vi "WFDC Get Current Drift.vi"(0 "Ref Images":T1[](array[typedef]), 2 "Z Calibration (slope, inter)":dbl[](array[numeric]), 5 "Half Shift":i32=7, 7 "Current Image":u16[][](array[numeric]), 11 "Error In":errorcluster, 13 "Track XY Drift?":bool=TRUE) -> (4 "Axis 1 Drift (px)":dbl, 6 "Axis 2 Drift (px)":dbl, 8 "Z Position (µm)":dbl format="%#_10g", 15 "Error Out":errorcluster)   [LabVIEW 2020]
uses:
  <vilib>/vision/Image Controls.llb/IMAQ Image.ctl
  WFDC DLL and Testing/Visual Studio NCC Max Shift DLL/x64/Release/VSmaxShiftNCC.dll
panel:
  out "Fit Middle Corr Image":dbl[][](graph)
  out "Middle Corr Image":dbl[][](graph)
  in  "Ref Image Pixel Size (µm)":dbl
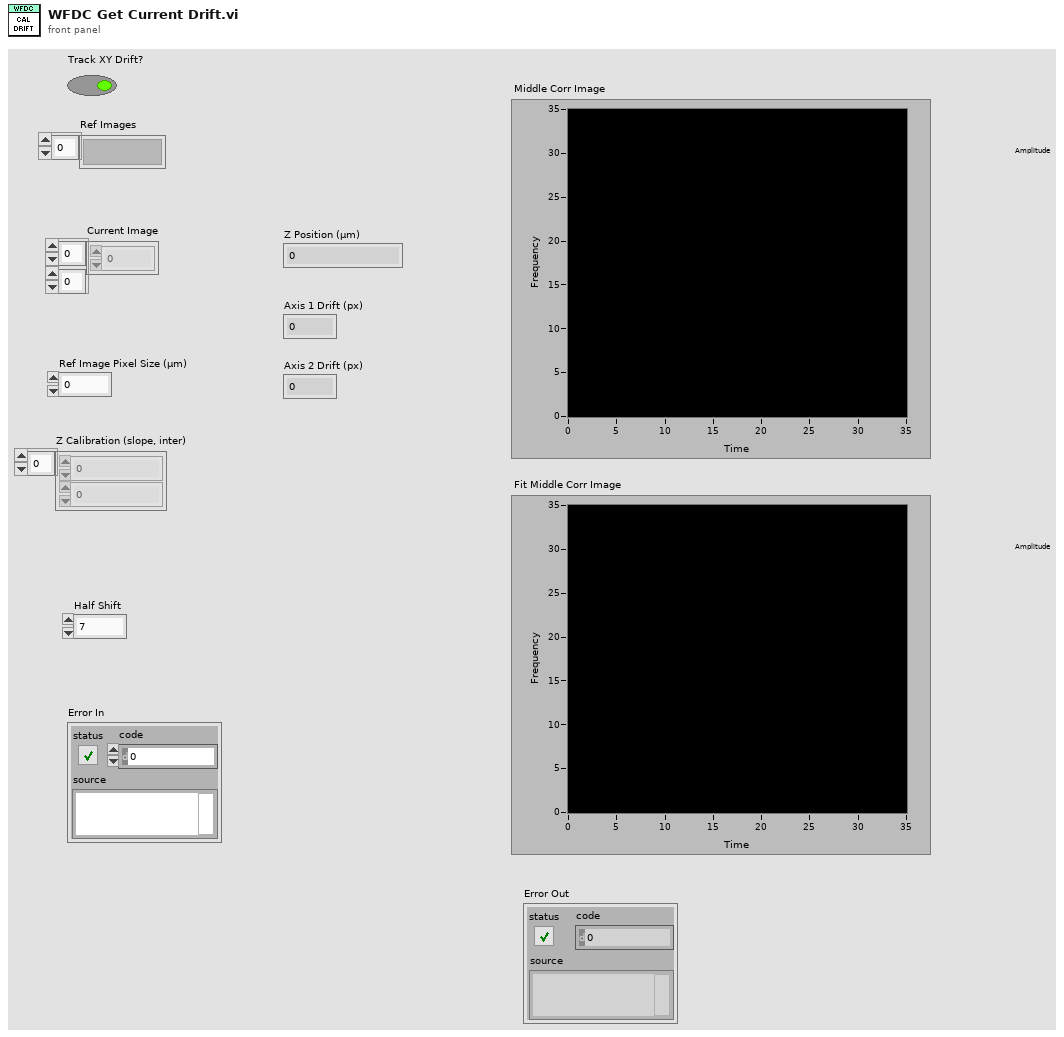
[diagram p1: front panel]
types:
  T1 = typedef "IMAQ Image.ctl" = refnum<image>
  T2 = typedef "2D Gaussian - Best Fit Parameters.ctl" = cluster{"Amplitude":dbl, "X Position":dbl, "Y Position":dbl, "X Width":dbl, "Y Width":dbl, "Offset":dbl}
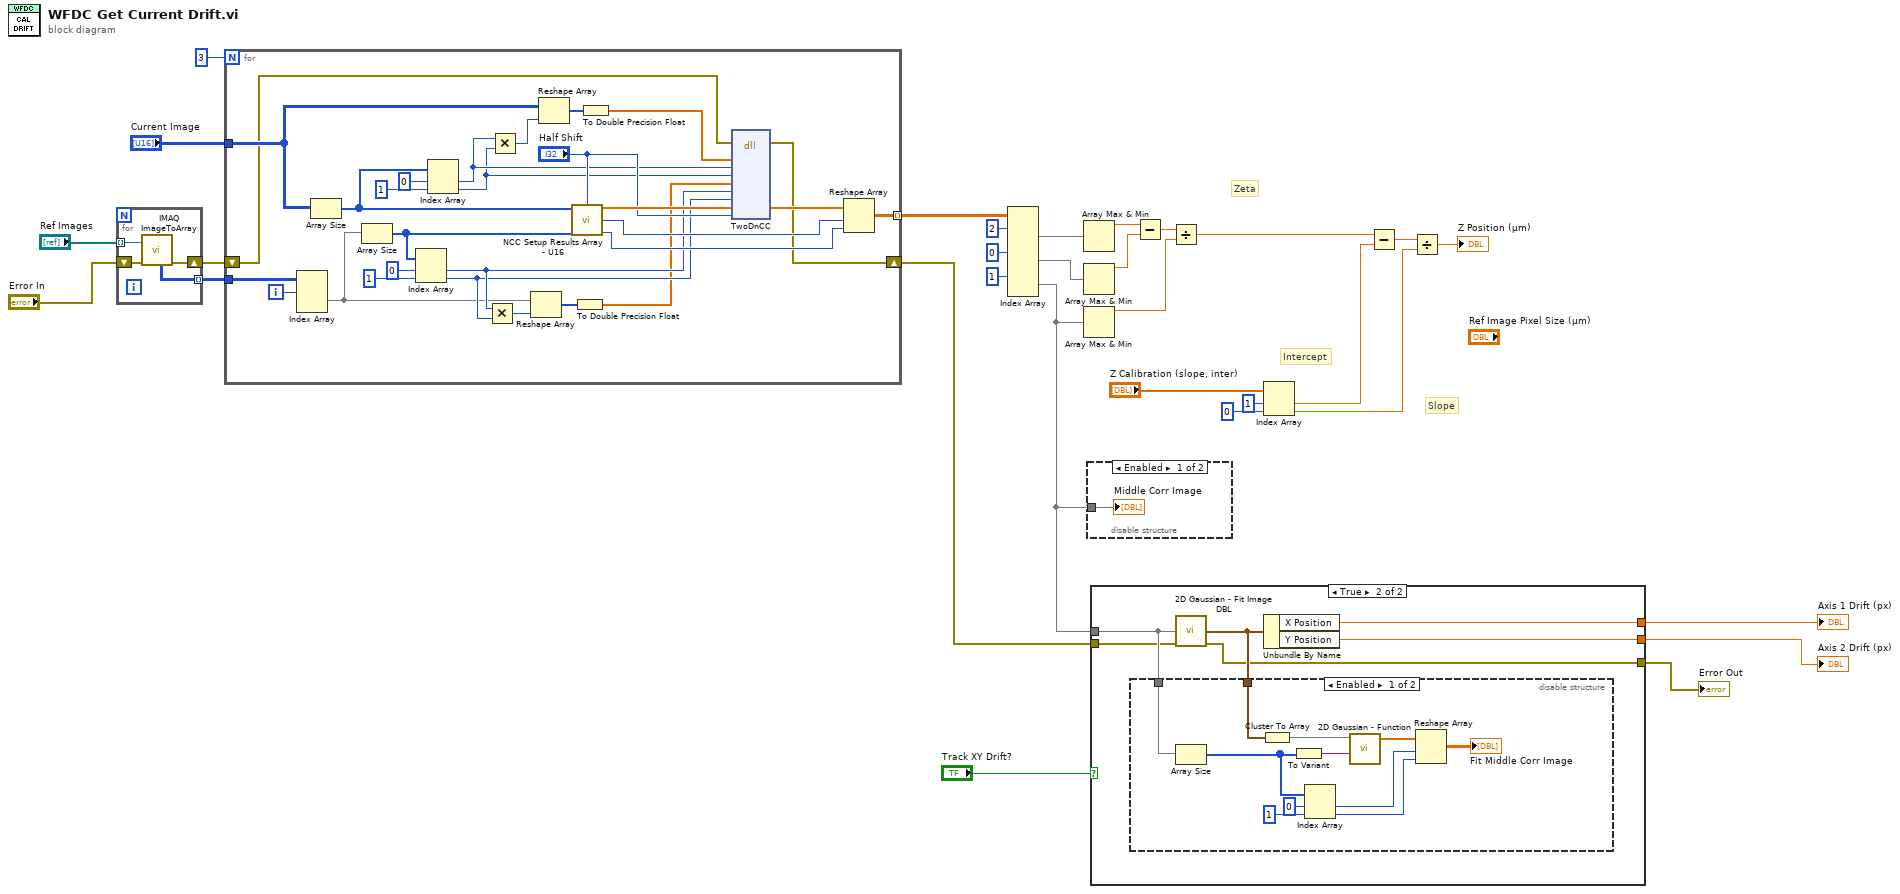
[diagram p0: block diagram]
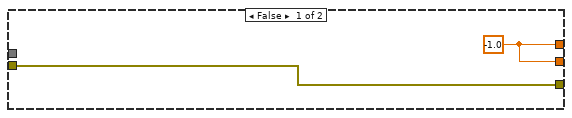
[diagram p2: hidden frame]
diagram:
  # "Slope"
  # "Zeta"
  # "Intercept"
  n1 = for {
    tunnel: "Ref Images" -> [w34] mode=indexing
    tunnel: [w33] -> w17 mode=indexing
    shift-right: [w31] -> w3
    shift-left: "Error In" -> [w32]
    n2 = call "IMAQ ImageToArray"("error in (no error)"=w32, "Image"=w34) -> ("Image Pixels (U16)"=w33:u16[][], "error out"=w31:errorcluster)  [unwired: 2 in, 3 out]
  }
  n3 = for {
    N: 3 -> [_]
    tunnel: w17 -> [w62]
    tunnel: "Current Image" -> [w42]
    tunnel: [w37] -> w29 mode=indexing
    shift-right: [w35] -> w2
    shift-left: w3 -> [w36]
    i -> [w61]
    n4 = Index Array(array=w62, index (dim 0)=w61) -> (element=w49:u16[][])  [unwired: 2 in]
    n5 = Array Size(array=w42) -> (size(s)=w44:i32[])
    n6 = Array Size(array=w49) -> (size(s)=w55:i32[])
    n7 = Index Array(array=w55, index #1=0 ("index"), index #2=1 ("index")) -> (element #1=w52:i32, element #2=w51:i32)
    n8 = Index Array(array=w44, index #1=0 ("index"), index #2=1 ("index")) -> (element #1=w40:i32, element #2=w39:i32)
    n9 = Multiply(x=w52, y=w51) -> (x*y=w50:i32)
    n10 = Multiply(x=w40, y=w39) -> (x*y=w38:i32)
    n11 = Reshape Array(w49, w50) -> (w48:u16[])
    n12 = Reshape Array(w42, w38) -> (w43:u16[])
    n13 = call "NCC Setup Results Array - U16.vi"("Image 01 Size"=w44, "Half Shift"="Half Shift", "Image 02 Size"=w55) -> ("NCC Results Array"=w60:dbl[], "Result Rows"=w57:i32, "Result Columns"=w58:i32)  [unwired: 10 in]
    n14 = To Double Precision Float(number=w48) -> (double precision float=w47:dbl[])
    n15 = To Double Precision Float(number=w43) -> (double precision float=w41:dbl[])
    n16 = dll-call lib="C:/Users/George Sirinakis/Documents/Microscope-Control/Microscope Modules/Wide Field Drift Correction/WFDC DLL and Testing/Visual Studio NCC Max Shift DLL/x64/Release/VSmaxShiftNCC.dll" fn="TwoDnCC"(error in=w36, "im01"=w41, "im01rowSize"=w40, "im01colSize"=w39, "im02"=w47, "im02rowSize"=w52, "im02ColSize"=w51, "theResult"=w60, "halfShift"="Half Shift") -> (error out=w35:errorcluster, "theResult"=w59:dbl[])  [unwired: 10 in, 1 out]
    n17 = Reshape Array(w59, w57, w58) -> (w37:dbl[][])
  }
  n18 = Index Array(array=w29, index (dim 0) #1=2 ("index (page)"), index (dim 0) #2=0 ("index (page)"), index (dim 0) #3=1 ("index (page)")) -> (element #1=w21:dbl[][], element #2=w20:dbl[][], element #3=w8:dbl[][])  [unwired: 6 in]
  n19 = Array Max & Min(array=w21) -> (max value=w25:dbl)  [unwired: 3 out]
  n20 = Array Max & Min(array=w20) -> (max value=w24:dbl)  [unwired: 3 out]
  n21 = Array Max & Min(array=w8) -> (max value=w22:dbl)  [unwired: 3 out]
  n22 = disable-structure shown="Enabled" {
    disable-tunnel: w8 -> [w63 _]
    frame Enabled {
      "Middle Corr Image" <- w63
    }
    frame Disabled {
    }
  }
  n23 = case shown="True" "Track XY Drift?" {
    tunnel: w8 -> [_ w69]
    tunnel: [w65 w71] -> w7
    tunnel: [w65 w70] -> w6
    tunnel: w2 -> [w64 w67]
    tunnel: [w64 w66] -> w1
    frame False {
      w65 = -1.0 ("X Position")
    }
    frame True {
      n24 = call "2D Gaussian - Fit Image DBL.vi"("Image In (DBL)"=w69, "Error In"=w67) -> ("Best Fit Params"=w68:T2, "Error Out"=w66:errorcluster)  [unwired: 12 in]
      n25 = disable-structure shown="Enabled" {
        disable-tunnel: w69 -> [w74 _]
        disable-tunnel: w68 -> [w73 _]
        frame Enabled {
          n26 = Array Size(array=w74) -> (size(s)=w78:i32[])
          n27 = Cluster To Array(cluster=w73) -> (array=w76:dbl[])
          n28 = To Variant(anything=w78) -> (Variant=w75:variant)
          n29 = Index Array(array=w78, index #1=0 ("index"), index #2=1 ("index")) -> (element #1=w81:i32, element #2=w82:i32)
          n30 = call "2D Gaussian - Function.vi"("data"=w75, "a"=w76) -> ("f(X,a)"=w77:dbl[])  [unwired: 2 in, 2 out]
          n31 = Reshape Array(w77, w81, w82) -> (→"Fit Middle Corr Image":dbl[][])
        }
        frame Disabled {
        }
      }
      n32 = Unbundle By Name(w68) -> ("X Position"=w71:dbl, "Y Position"=w70:dbl)
    }
  }
  "Axis 2 Drift (px)" <- w6
  "Axis 1 Drift (px)" <- w7
  "Error Out" <- w1
  n33 = Subtract(x=w25, y=w24) -> (x-y=w23:dbl)
  n34 = Divide(x=w23, y=w22) -> (x/y=w13:dbl)
  n35 = Index Array(array="Z Calibration (slope, inter)", index #1=1 ("index"), index #2=0 ("index")) -> (element #1=w12:dbl, element #2=w10:dbl)
  n36 = Subtract(x=w13, y=w12) -> (x-y=w11:dbl)
  n37 = Divide(x=w11, y=w10) -> (x/y=→"Z Position (µm)":dbl)
